vi "Bridge Sim Null Xfer.vi"(0 "f [Hz]":dbl format="%#_6p") -> (5 "aperture":dbl, 6 "gain":dbl format="%#_6p", 8 "phi":dbl format="%#_6p", 9 "fs":dbl)   [LabVIEW 2013]
doc: "Simulate zero transfer measurement for digitizer correction generation (connected U-I channels)."
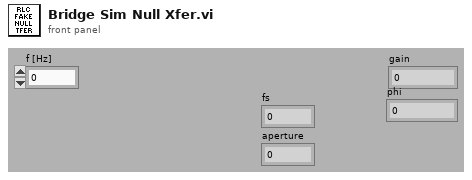
[diagram p1: front panel]
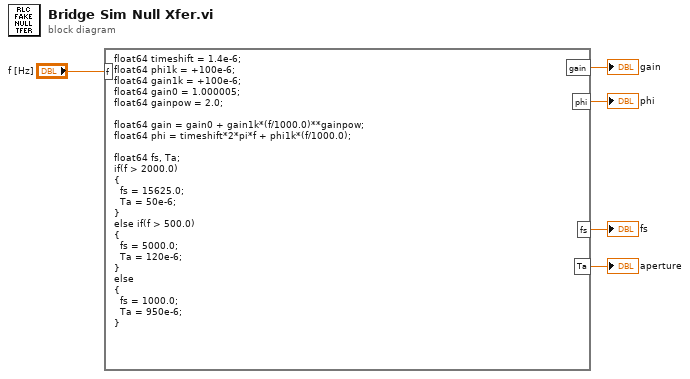
[diagram p0: block diagram]
diagram:
  n1 = formula code="float64 timeshift = 1.4e-6;\nfloat64 phi1k = +100e-6;\nfloat64 gain1k = +100e-6;\nfloat64 gain0 = 1.000005;\nfloat64 gainpow = 2.0;\n\nfloat64 gain = gain0 + gain1k*(f/1000.0)**gainpow;\nfloat64 phi = timeshift*2*pi*f + phi1k*(f/1000.0);\n\nfloat64 fs, Ta;\nif(f > 2000.0)\n{\n  fs = 15625.0;\n  Ta = 50e-6;\n}\nelse if(f > 500.0)\n{\n  fs = 5000.0;\n  Ta = 120e-6;\n}\nelse\n{\n  fs = 1000.0;\n  Ta = 950e-6;\n}"("f"="f [Hz]") -> ("gain"=→"gain":dbl, "phi"=→"phi":dbl, "fs"=→"fs":dbl, "Ta"=→"aperture":dbl)
